vi "PI_MoveTo.vi"(0 "System no.":i32, 2 "Target position":dbl[](array[numeric]), 5 "error in":errorcluster, 6 "Move":bool) -> (14 "System no. (dup)":i32, 16 "Position":dbl[](array[numeric]), 19 "error out":errorcluster)   [LabVIEW 2013]
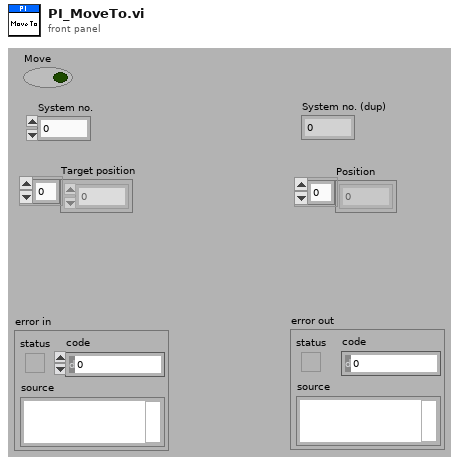
[diagram p1: front panel]
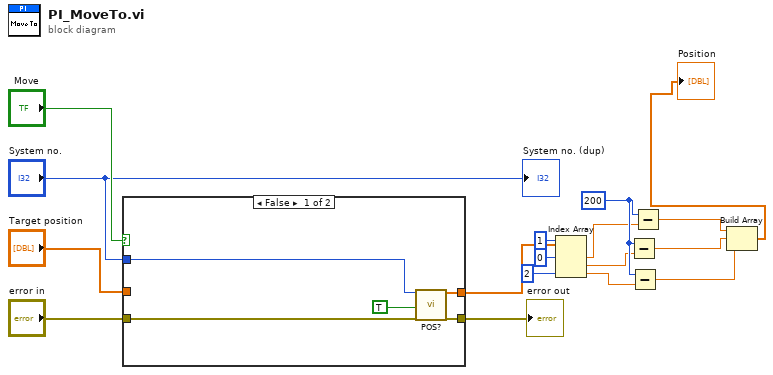
[diagram p0: block diagram]
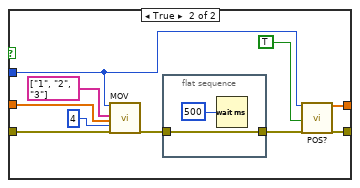
[diagram p2: hidden frame]
diagram:
  w12 = 200
  n1 = case shown="False" "Move" {
    tunnel: [w22 w27] -> w17
    tunnel: "error in" -> [w20 w32]
    tunnel: "System no." -> [w19 w26]
    tunnel: [w18 w25] -> w11
    tunnel: "Target position" -> [_ w30]
    frame False {
      n2 = call "POS?.vi"("System no."=w19, "All axes?"=TRUE, "error in"=w20) -> ("Position"=w18:dbl[], "error out"=w22:errorcluster)  [unwired: 2 in, 13 out]
    }
    frame True {
      n3 = call "MOV.vi"("System no."=w26, "Axes to move"=string[] ["1", "2", "3"], "Position values"=w30, "No.of digits"=i16 4, "error in"=w32) -> ("error out"=w24:errorcluster)  [unwired: 14 in]
      n4 = flat-sequence {
        tunnel: w24 -> [w34]
        tunnel: [w34] -> w23
        frame #0 {
          n5 = Wait (ms)(milliseconds to wait=u32 500) -> ()  [unwired: 1 out]
        }
      }
      n6 = call "POS?.vi"("System no."=w26, "All axes?"=TRUE, "error in"=w23) -> ("Position"=w25:dbl[], "error out"=w27:errorcluster)  [unwired: 15 in]
    }
  }
  "error out" <- w17
  n7 = Index Array(array=w11, index #1=0 ("index"), index #2=1 ("index"), index #3=2 ("index")) -> (element #1=w7:dbl, element #2=w6:dbl, element #3=w5:dbl)
  n8 = Subtract(x=w12, y=w6) -> (x-y=w3:dbl)
  n9 = Subtract(x=w12, y=w5) -> (x-y=w2:dbl)
  n10 = Subtract(x=w12, y=w7) -> (x-y=w4:dbl)
  n11 = Build Array(w4, w3, w2) -> (→"Position":dbl[])
  "System no. (dup)" <- "System no."
